vi "View.vi"(8 "error in (no error)":errorcluster, 11 "View In":refnum<class "View.lvclass">) -> (0 "error out":errorcluster, 3 "View Out":refnum<class "View.lvclass">)   [LabVIEW 2020, in "View.lvclass"]
doc: "This VI implements the main UI of the process. A reference to this VI should be set using the Set View VI Reference.vi method when the VI is started."
uses:
  View.lvclass
  C:/Users/anton/Documents/GitHub/Triarc-Framework/source/Framework/Process/Process.lvclass
  View.lvclass/View.ctl
  Process/Process.lvclass/Process.ctl
  Process/Process.lvclass
  Error Handler Interface/Error Handler Interface.lvclass
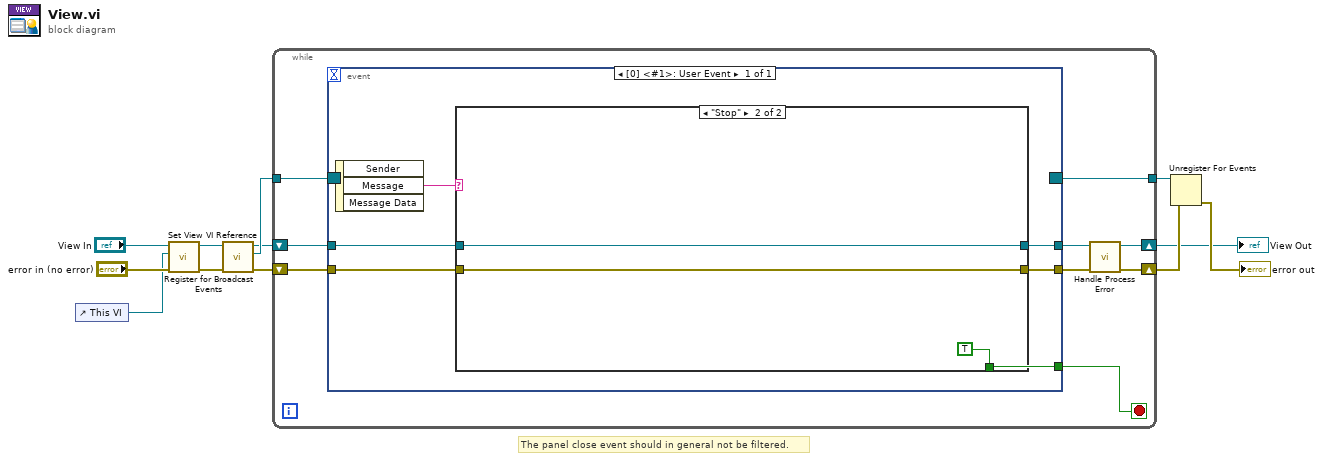
[diagram p0: block diagram]
diagram:
  # "The panel close event should in general not be filtered."
  n1 = control-ref of="This VI"() -> (w1:refnum<vi>)
  n2 = call "Set View VI Reference.vi"("error in (no error)"="error in (no error)", "View VI Reference"=w1, "UI View in"="View In") -> ("error out"=w2:errorcluster, "UI View out"=w4:refnum<class "View.lvclass">)  [unwired: 7 in]
  n3 = call-dynamic "Register for Broadcast Events.vi"("error in (no error)"=w2, "Process In"=w4) -> ("error out"=w8:errorcluster, "Event Registration Refnum"=w12:refnum<event-registration>, "Process Out"=w9:refnum<class "View.lvclass">)  [unwired: 7 in]
  n4 = while {
    shift-right: [w15] -> w6
    shift-left: w9 -> [w21]
    shift-right: [w13] -> w10
    shift-left: w8 -> [w19]
    tunnel: w12 -> [w18]
    tunnel: [w17] -> w11
    stop <- w16 stop-if-true
    n5 = event shown="[0] <#1>: User Event" {
      selector: w18 -> [_]
      dyn-events: [_] -> w17
      timeout: _ -> [_]
      tunnel: w21 -> [w27]
      tunnel: [w26] -> w20
      tunnel: w19 -> [w24]
      tunnel: [w25] -> w14
      tunnel: [w22] -> w16
      event User Event {
        n6 = event-data() -> ("Message"=w23:string)  [unwired: 1 in, 2 out]
        n7 = case shown="\"Stop\"" w23 {
          tunnel: w27 -> [w29 w32]
          tunnel: [w29 w32] -> w26
          tunnel: [w28 w31] -> w25
          tunnel: w24 -> [w28 w31]
          tunnel: [_ TRUE] -> w22
          frame Default {
          }
          frame "Stop" {
          }
        }
      }
    }
    n8 = call "Handle Process Error.vi"("error in (no error)"=w14, "Process In"=w20) -> ("error out"=w13:errorcluster, "Process Out"=w15:refnum<class "View.lvclass">)  [unwired: 8 in]
  }
  "View Out" <- w6
  n9 = Unregister For Events(event registration refnum=w11, error in=w10) -> (error out=→"error out":errorcluster)
